vi "light_setRange.vi"(9 "error in (no error)":errorcluster, 10 "Visa Session":refnum<visa-resource-name>="USB0::0x0BD3::0x0333::NI-VISA-30004::RAW", 11 "range":T1(ring)) -> (1 "Device Response":string="*\n", 2 "dup Visa Session":refnum<visa-resource-name>="USB0::0x0BD3::0x0333::NI-VISA-30004::RAW", 8 "error out":errorcluster)   [LabVIEW 2018]
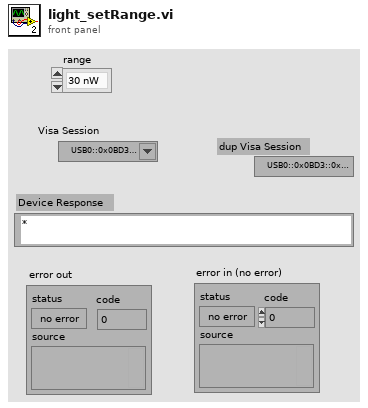
[diagram p1: front panel]
types:
  T1 = enum16{"30 nW", "300 nW", "3 uW", "300 uW", "AUTO", "30 mW", "3 mW", "30 uW"}
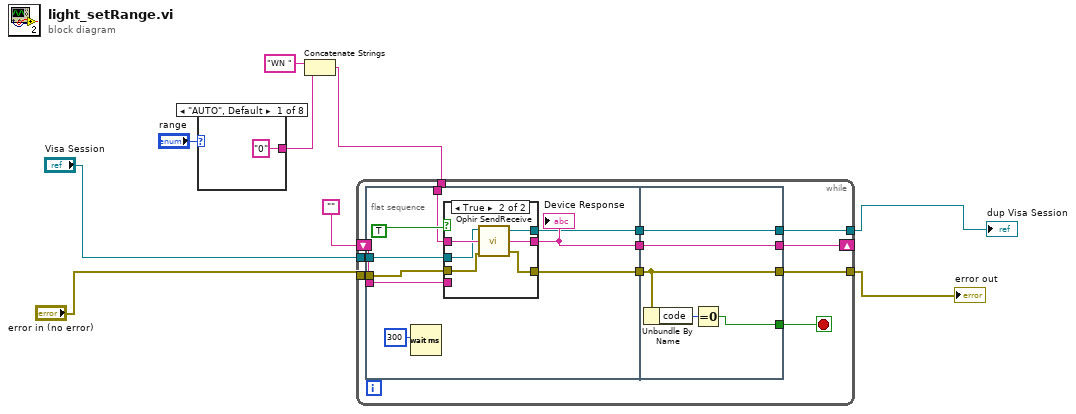
[diagram p0: block diagram]
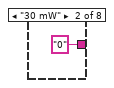
[diagram p2: hidden frame]
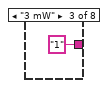
[diagram p3: hidden frame]
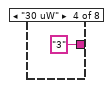
[diagram p4: hidden frame]
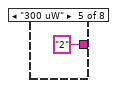
[diagram p5: hidden frame]
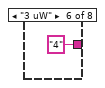
[diagram p6: hidden frame]
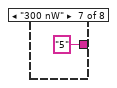
[diagram p7: hidden frame]
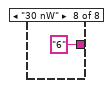
[diagram p8: hidden frame]
diagram:
  n1 = case shown="\"AUTO\", Default" "range" {
    tunnel: ["0" ("wave nm") "0" ("wave nm") "1" ("wave nm") "3" ("wave nm") "2" ("wave nm") "4" ("wave nm") "5" ("wave nm") "6" ("wave nm")] -> w2
    frame "AUTO", Default {
    }
    frame "30 mW" {
    }
    frame "3 mW" {
    }
    frame "30 uW" {
    }
    frame "300 uW" {
    }
    frame "3 uW" {
    }
    frame "300 nW" {
    }
    frame "30 nW" {
    }
  }
  n2 = Concatenate Strings("WN " ("string"), w2) -> (w4:string)
  n3 = while {
    tunnel: [w25] -> w6
    tunnel: [w23] -> w8
    shift-left: "" -> [w27]
    shift-right: [w28] -> _
    tunnel: "error in (no error)" -> [w24]
    tunnel: "Visa Session" -> [w26]
    tunnel: w4 -> [w22]
    stop <- w18 stop-if-true
    n4 = flat-sequence {
      tunnel: w27 -> [w35]
      tunnel: w26 -> [w34]
      tunnel: w24 -> [w31]
      tunnel: w22 -> [w29]
      tunnel: [w36] -> w21
      tunnel: [w33] -> w20
      tunnel: [w30] -> w19
      tunnel: [w48] -> w23
      tunnel: [w50] -> w25
      tunnel: [w51] -> w28
      tunnel: w21 -> [w51]
      tunnel: w20 -> [w50]
      tunnel: w19 -> [w48]
      tunnel: [w47] -> w18
      frame #0 {
        n5 = Wait (ms)(milliseconds to wait=u32 300) -> ()  [unwired: 1 out]
        n6 = case shown="True" TRUE ("Send Command (Enter)") {
          tunnel: w29 -> [_ w46]
          tunnel: [w40 w45] -> w36
          tunnel: w35 -> [w40 _]
          tunnel: w34 -> [w39 w44]
          tunnel: w31 -> [w38 w43]
          tunnel: [w38 w42] -> w30
          tunnel: [w39 w41] -> w33
          frame False {
          }
          frame True {
            n7 = call "Ophir SendReceive.vi"("error in (no error)"=w43, "Command"=w46, "Visa Session"=w44) -> ("error out"=w42:errorcluster, "Frame Output"=w45:string, "dup Visa Session"=w41:refnum<visa-resource-name>)
          }
        }
        "Device Response" <- w36
      }
      frame #1 {
        n8 = Unbundle By Name(w48) -> ("code"=w49:i32)
        n9 = Equal To 0?(x=w49) -> (x = 0?=w47:bool)
      }
    }
  }
  "error out" <- w8
  "dup Visa Session" <- w6
